vi "attoCall_DLL.vi"(8 "error in":errorcluster, 9 "params":string="1", 10 "method":string="com.attocube.amc.control.getActorName", 11 "deviceHandle":i32) -> (0 "error out":errorcluster, 2 "response":string, 3 "deviceHandle out":i32)   [LabVIEW 2016]
uses:
  Release/LabVIEWJSON.dll
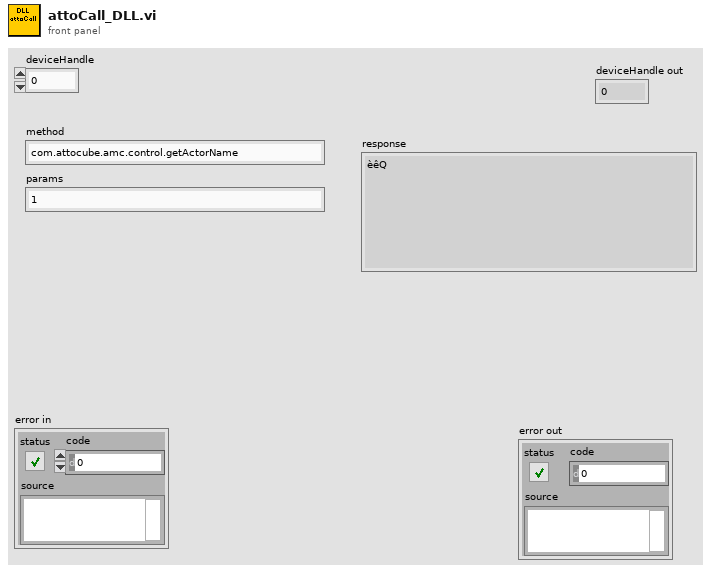
[diagram p1: front panel]
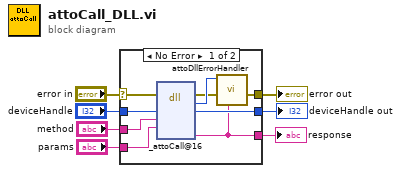
[diagram p0: block diagram]
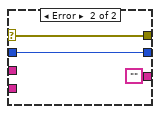
[diagram p2: hidden frame]
diagram:
  n1 = case shown="No Error" "error in" {
    selector: "error in" -> [w11 w19]
    tunnel: [w8 ""] -> w7
    tunnel: "deviceHandle" -> [w14 w18]
    tunnel: [w13 w18] -> w1
    tunnel: [w12 w19] -> w2
    tunnel: "method" -> [w10 _]
    tunnel: "params" -> [w9 _]
    frame No Error {
      n2 = dll-call lib="C:/Users/schieda/OneDrive - WITTENSTEIN SE/Desktop/LabVIEW/API_Autogen_v1.3_DSc/generatedAPIs/AMC_VIs_DLL (for older LV Versions only)/DLLHandler/Release/LabVIEWJSON.dll" fn="_attoCall@16"(error in=w11, "deviceHandle"=w14, "method"=w10, "params"=w9) -> (error out=w15:errorcluster, "rc"=w16:i32, "deviceHandle"=w13:i32, "response"=w8:string)  [unwired: 5 in, 1 out]
      n3 = call "attoDllErrorHandler.vi"("response"=w8, "error in"=w15, "rc"=w16) -> ("error out"=w12:errorcluster)  [unwired: 8 in]
    }
    frame Error {
    }
  }
  "response" <- w7
  "error out" <- w2
  "deviceHandle out" <- w1
